vi "Config Path--constant.vi"() -> (3 "File Path":path=path "C:/Users/AlexPai/Desktop/config data")   [LabVIEW 2020, in "CML Shared.lvlib"]
uses:
  CML Shared.lvlib
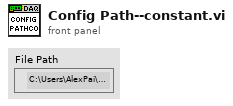
[diagram p1: front panel]
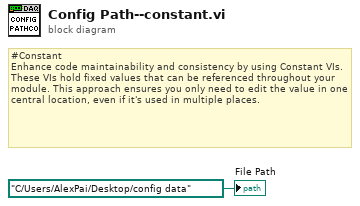
[diagram p0: block diagram]
diagram:
  # "#Constant\nEnhance code maintainability and consistency by using Constant VIs. These VIs hold fixed values that can be referenced throughout your module. This approach ensures you only need to edit the value in one central location, even if it's used in multiple places."
  "File Path" <- path "C:/Users/AlexPai/Desktop/config data" ("File Path")
